vi "main.vi"() -> ()   [LabVIEW 2014]
panel:
  out "Total count":i32
  out "Count 2":i32
  out "running totaL":i32
  out "Count 1":i32
  in  "Stop":bool
  out "running total":i32
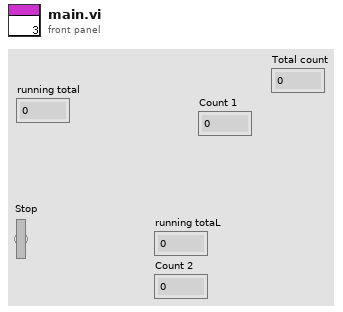
[diagram p1: front panel]
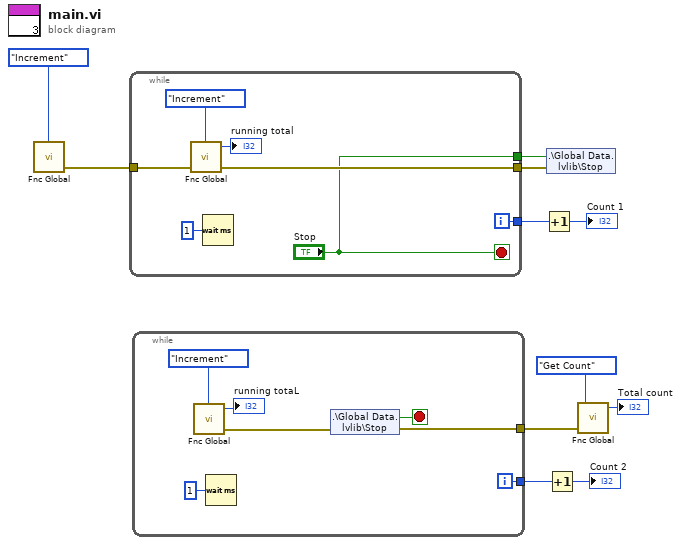
[diagram p0: block diagram]
diagram:
  n1 = call "Fnc Global.vi"("Command"=enum8{"Increment", "Reset", "Get Count"}."Increment") -> ("error out"=w10:errorcluster)  [unwired: 3 in, 1 out]
  n2 = while {
    tunnel: w10 -> [w17]
    tunnel: [w16] -> w9
    tunnel: ["Stop"] -> w8
    tunnel: [w12] -> w7
    i -> [w12]
    stop <- "Stop" stop-if-true
    n3 = call "Fnc Global.vi"("error in (no error)"=w17, "Command"=enum8{"Increment", "Reset", "Get Count"}."Increment") -> ("error out"=w16:errorcluster, "Numeric"=→"running total":i32)  [unwired: 2 in]
    n4 = Wait (ms)(milliseconds to wait=u32 1) -> ()  [unwired: 1 out]
  }
  n5 = while {
    tunnel: [w22] -> w5
    tunnel: [w20] -> w3
    i -> [w22]
    stop <- w19 stop-if-true
    n6 = call "Fnc Global.vi"("Command"=enum8{"Increment", "Reset", "Get Count"}."Increment") -> ("error out"=w21:errorcluster, "Numeric"=→"running totaL":i32)  [unwired: 3 in]
    n7 = Wait (ms)(milliseconds to wait=u32 1) -> ()  [unwired: 1 out]
    n8 = shared-variable ".\\Global Data.lvlib\\Stop"(error in=w21) -> (w19:bool, error out=w20:errorcluster)
  }
  n9 = Increment(x=w7) -> (x+1=→"Count 1":i32)
  n10 = shared-variable ".\\Global Data.lvlib\\Stop"(w8, error in=w9) -> ()  [unwired: 1 out]
  n11 = Increment(x=w5) -> (x+1=→"Count 2":i32)
  n12 = call "Fnc Global.vi"("error in (no error)"=w3, "Command"=enum8{"Increment", "Reset", "Get Count"}."Get Count") -> ("Numeric"=→"Total count":i32)  [unwired: 2 in, 1 out]
